vi "set_QWP.vi"(1 "Quarter Wave Plate":T1={"QWP"=TRUE, "QWP angles"="", "reverse"=TRUE}) -> (0 "Tot QWP Arr":dbl[](array[numeric]))   [LabVIEW 2018]
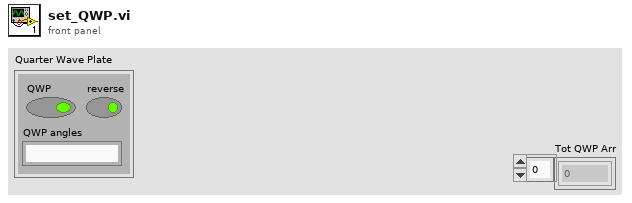
[diagram p1: front panel]
types:
  T1 = cluster{"QWP":bool, "QWP angles":string, "reverse":bool}
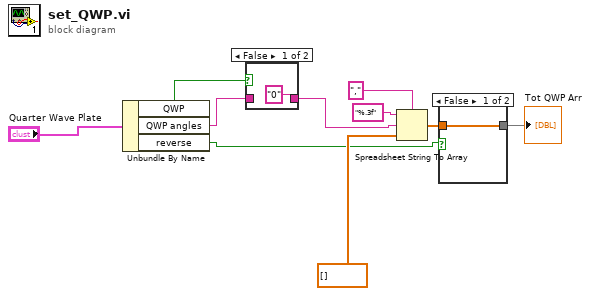
[diagram p0: block diagram]
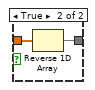
[diagram p3: hidden frame]
diagram:
  n1 = Unbundle By Name("Quarter Wave Plate") -> ("QWP"=w1:bool, "QWP angles"=w3:string, "reverse"=w6:bool)
  n2 = case shown="False" w1 {
    tunnel: w3 -> [_ w12]
    tunnel: ["0" ("QWP angles") w12] -> w2
    frame False {
    }
    frame True {
    }
  }
  n3 = Spreadsheet String To Array(delimiter (Tab)=",", format string="%.3f", spreadsheet string=w2, array type (2D Dbl)=dbl[] []) -> (array=w5:dbl[])
  n4 = case shown="False" w6 {
    tunnel: w5 -> [w13 w15]
    tunnel: [w13 w14] -> w4
    frame False {
    }
    frame True {
      n5 = Reverse 1D Array(array=w15) -> (reversed array=w14:dbl[])
    }
  }
  "Tot QWP Arr" <- w4
